vi "Multi RefTriggerScope with digital read long run.vi"() -> ()   [LabVIEW 2023]
uses:
  RefTriggerApplication/ApplicationCluster.ctl
  <instrlib>/niScope/Controls/niScope trigger source digital.ctl
  <instrlib>/niScope/Controls/niScope trigger slope.ctl
  <instrlib>/niDigital/niDigital.llb/niDigital Export Signal.ctl
  <instrlib>/niDigital/niDigital.llb/niDigital Trigger Digital Edge - Edge.ctl
  <instrlib>/niDigital/niDigital.llb/niDigital Trigger Terminals.ctl
  <instrlib>/niDCPower/nidcpower.llb/niDCPower Export Signal - Signal.ctl
  <instrlib>/niDCPower/nidcpower.llb/niDCPower Wait For Event - Event.ctl
  <instrlib>/niScope/Configure/Trigger/niScope Configure Trigger Digital.vi
  <instrlib>/niDigital/niDigital.llb/niDigital Disable Start Trigger.vi
  <instrlib>/niDigital/niDigital.llb/niDigital Write Source Waveform (Broadcast U32).vi
  <instrlib>/niDigital/niDigital.llb/niDigital Configure Digital Edge Start Trigger.vi
  <instrlib>/niScope/Acquire/Fetch/niScope Fetch.vi
  <vilib>/Utility/file.llb/Write Delimited Spreadsheet (DBL).vi
  <instrlib>/NIDigital Low-Level SPI/NIDigital Low-Level SPI.lvclass
  <instrlib>/niDigital/niDigital.llb/niDigital Burst Pattern (Pass Fail).vi
panel:
  in  "LoggingPath":path
  in  "Stop":bool
  out "SMU":dbl[](graph)
  in  "Trigger Through":enum16{"DigitalPattern", "SMU"}(ring)
  in  "Instrument Settings":enum32{"SMU", "Scope", "Digital Pattern"}(tab)
  in  "SMU name":refnum<k15>
  in  "Scope Name 2":refnum<k15>="Scope_5152_C02_S05" caption="Scope  Name(s)"
  in  "Scope Name":refnum<k15>="Scope_5152_C02_S05" caption="Scope  Name(s)"
  in  "Sample Rate":dbl=5000000.0 format="%#.2p"
  in  "Record Length":i32=10000 format="%.0p"
  in  "Reference Position":dbl=50.0 caption="Ref Position" format="%#.1f"
  in  "DigiPat name":refnum<k15>
  in  "pin list":string="SCLK_SPI, MOSI_SPI, MISO_SPI, CS_SPI"
  out "Scope":dbl[][](graph)
  out "Digital Data":u32[][](array[numeric]) format="%.0x"
  out "error out":errorcluster
  in  "error in":errorcluster
  # "SDA"
  # "Other pin"
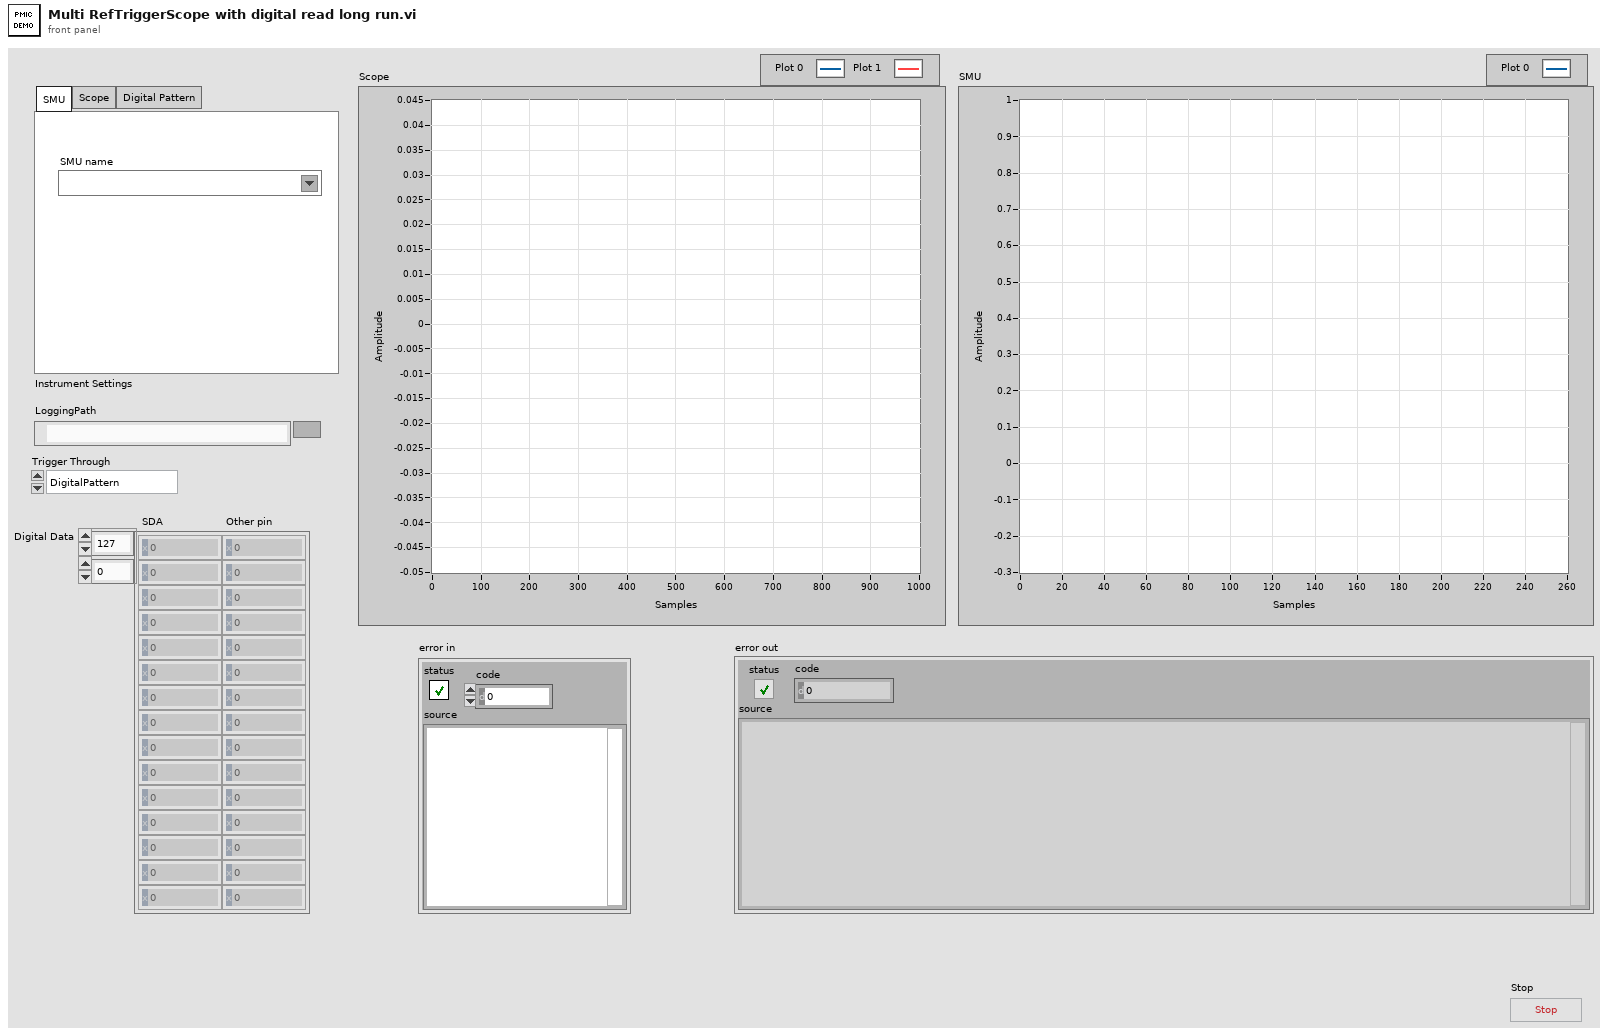
[diagram p1: front panel]
types:
  T1 = typedef "ApplicationCluster.ctl" = cluster{"Scope Name":refnum<k15>, "Scope channel name":string, "DigiPat name":refnum<k15>, "pin list":string, "DigitalWaveformName":string, "DigitalData":u32[][], "SMU name":refnum<k15>, "SMU Channel Name":string, "SMU Sequence Name":string, "Scope wfm":dbl[][], "SMU wfv":dbl[], "Record Length Scope":i32, "Scope Name 2":refnum<k15>, "Scope channel name 2":string}
  T2 = cluster{"Digital Data":u32[][], "SMU wfv":dbl[], "Scope wfm":dbl[][]}
  T3 = typedef "niScope trigger source digital.ctl" = string
  T4 = typedef "niDigital Trigger Terminals.ctl" = string
  T5 = typedef "niScope trigger slope.ctl" = i32
  T6 = typedef "niDigital Export Signal.ctl" = i32
  T7 = typedef "niDCPower Export Signal - Signal.ctl" = i32
  T8 = typedef "niDigital Trigger Digital Edge - Edge.ctl" = i32
  T9 = typedef "niDCPower Wait For Event - Event.ctl" = i32
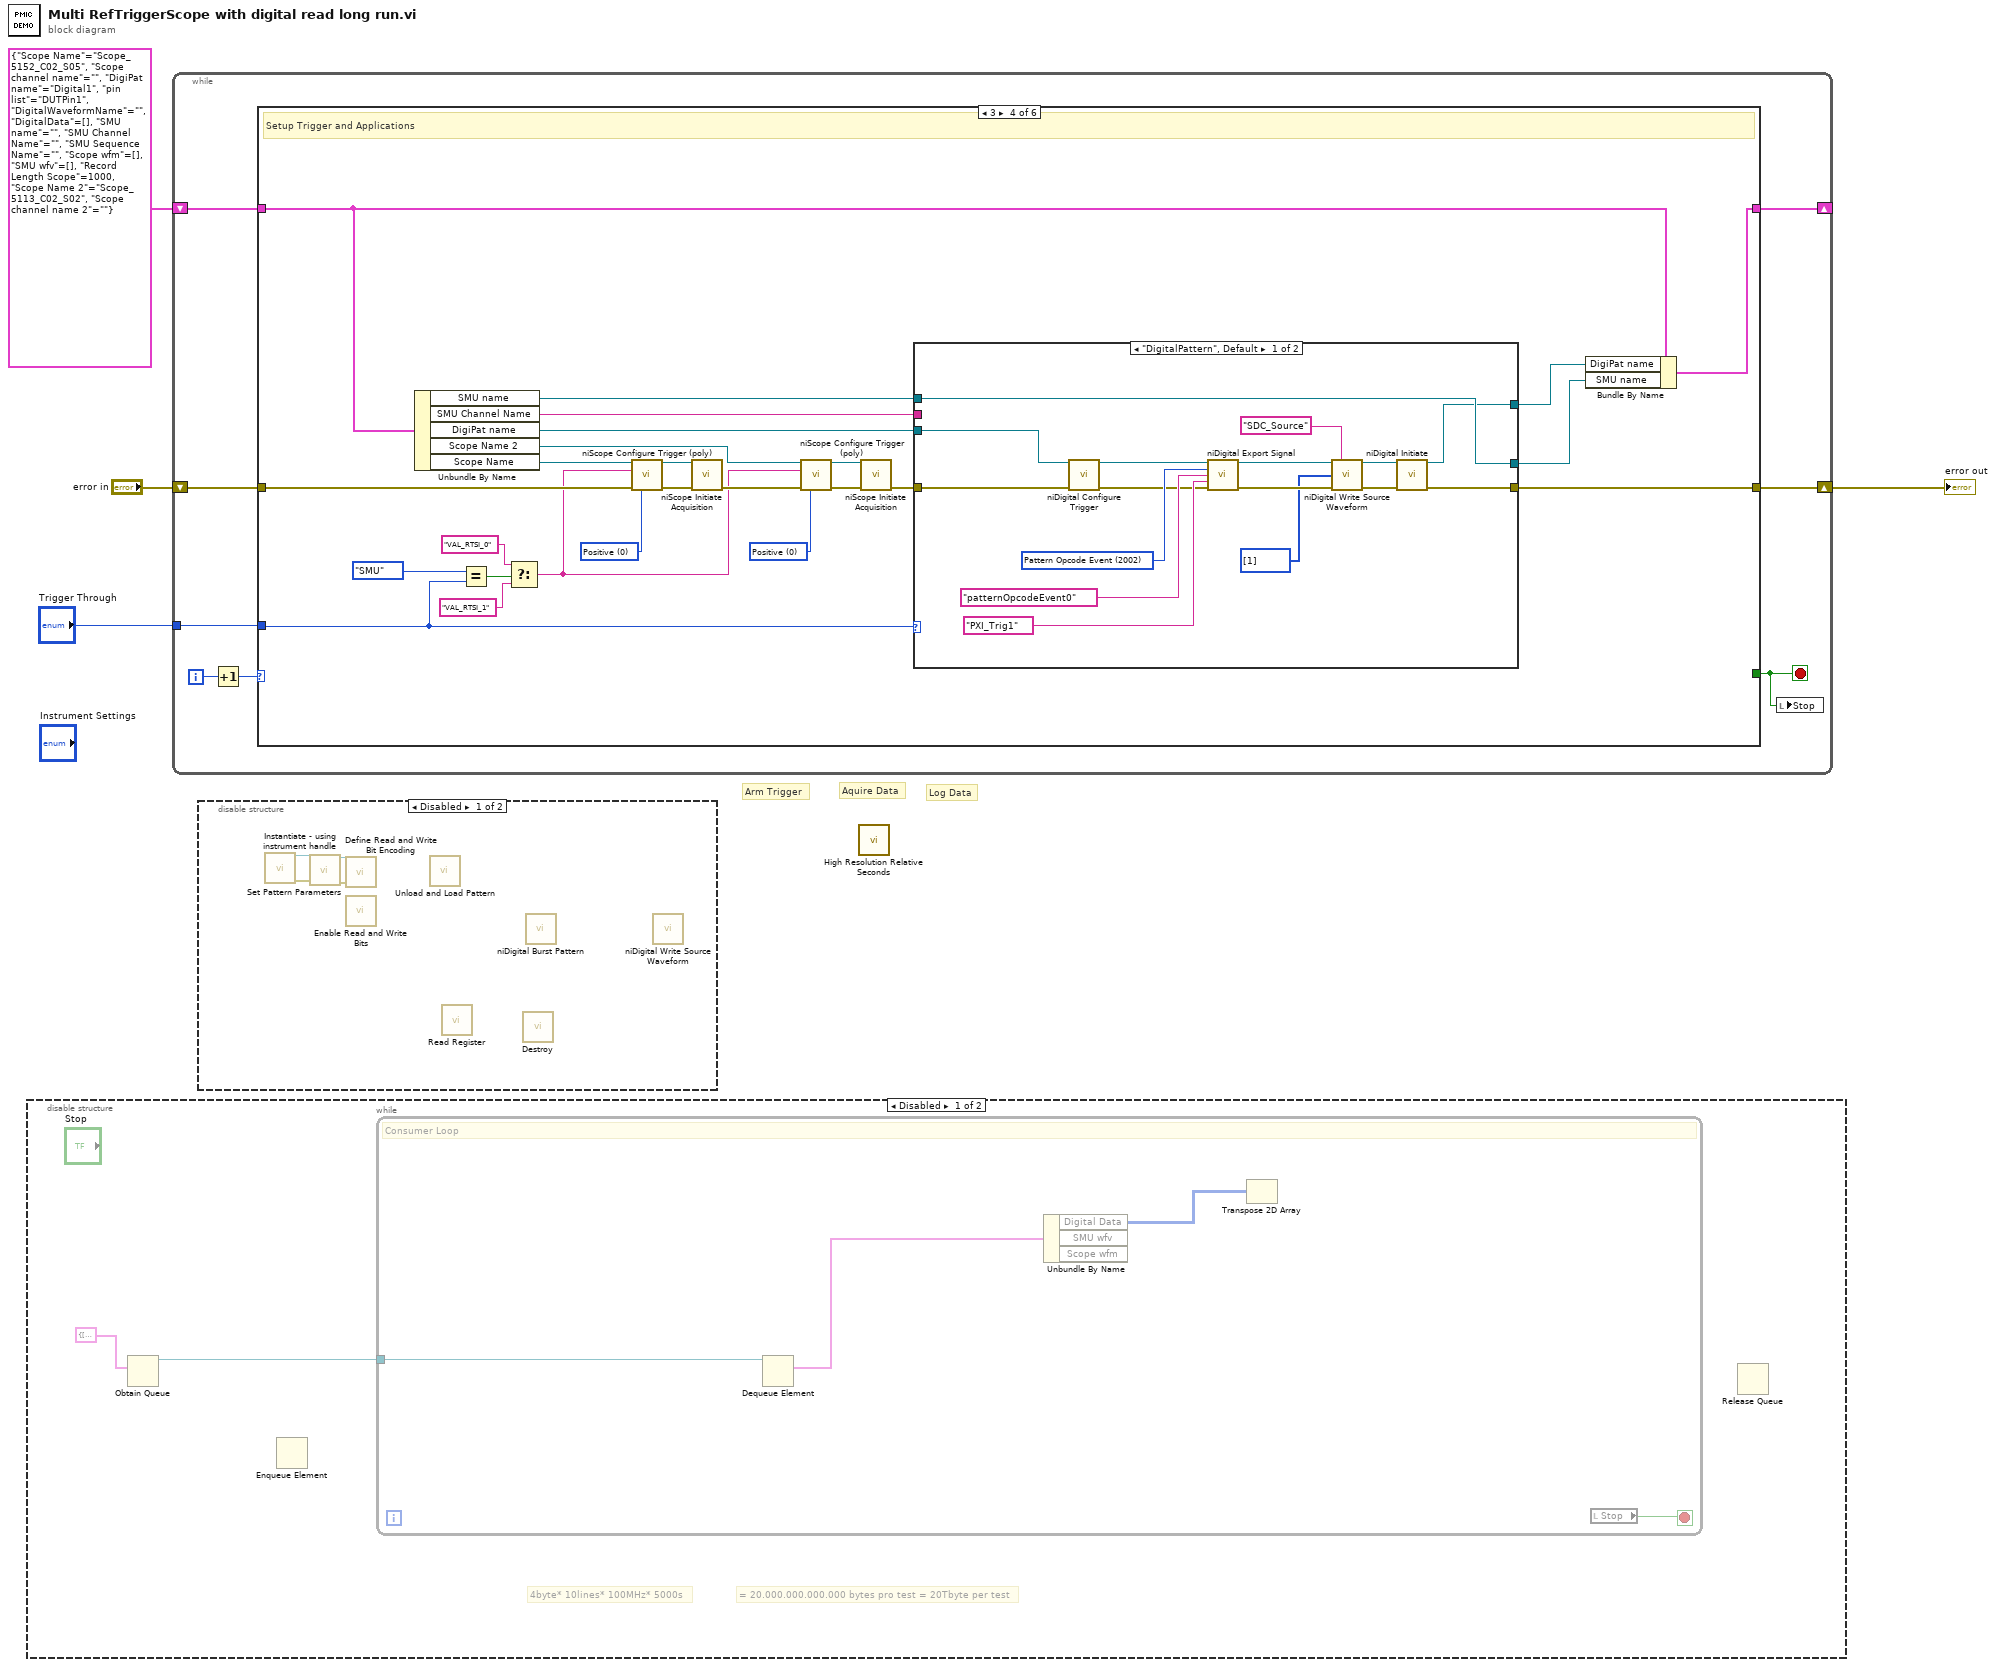
[diagram p0: block diagram]
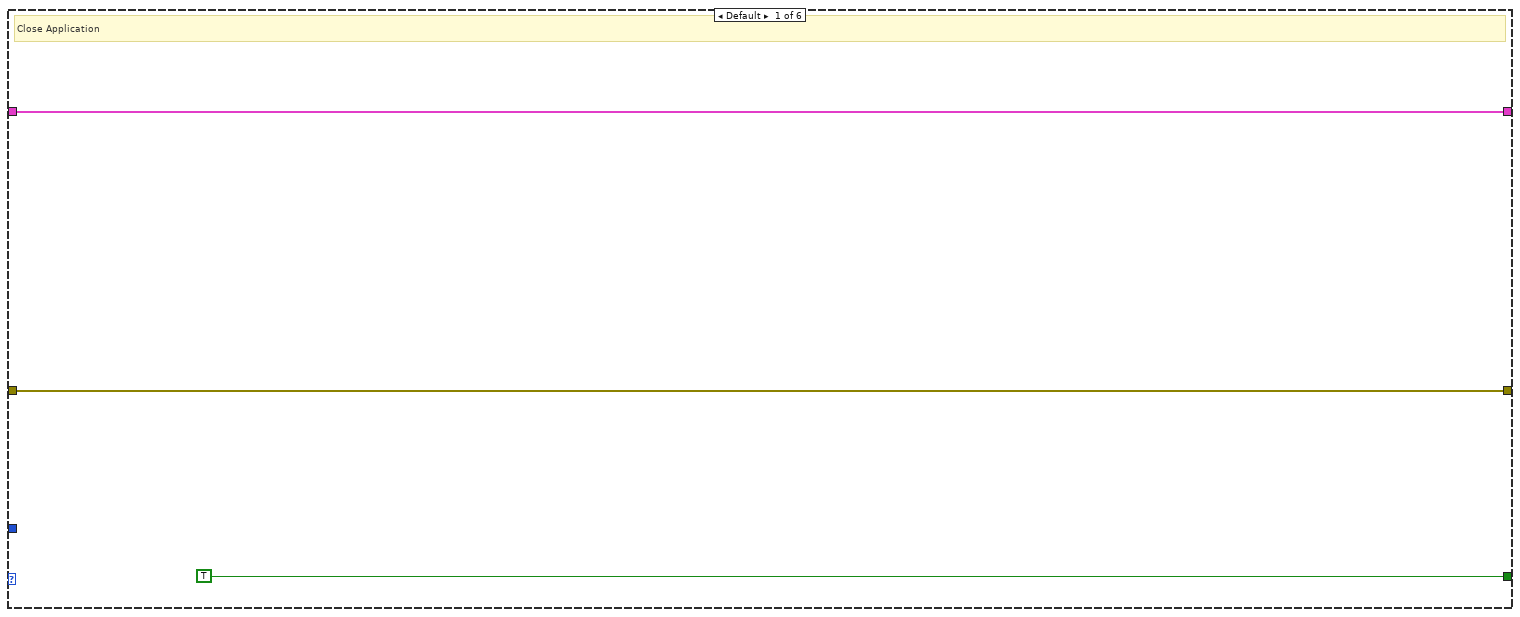
[diagram p4: hidden frame]
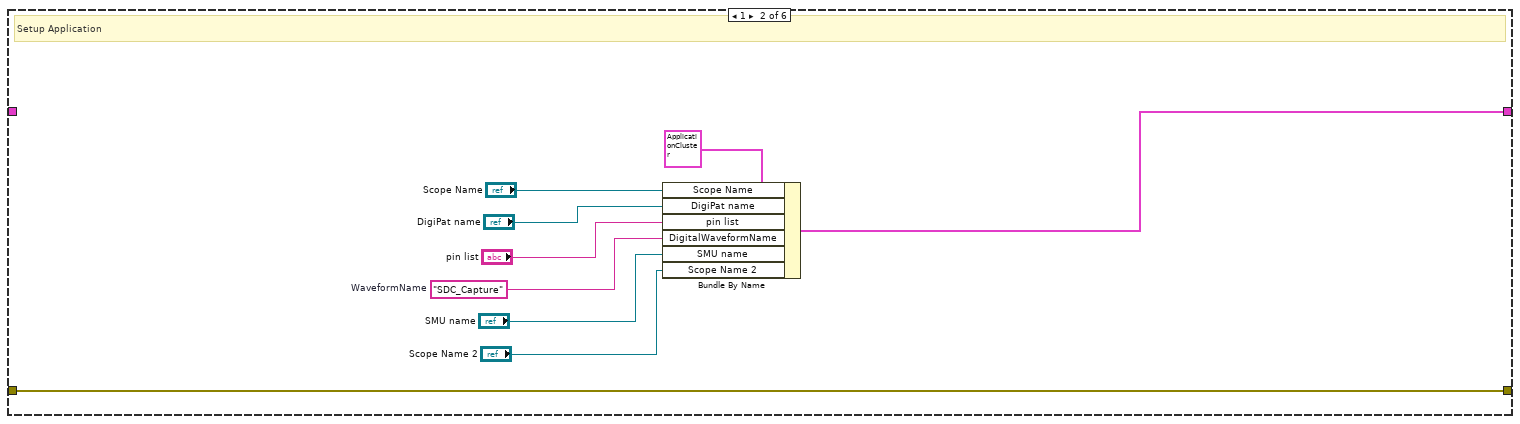
[diagram p5: hidden frame]
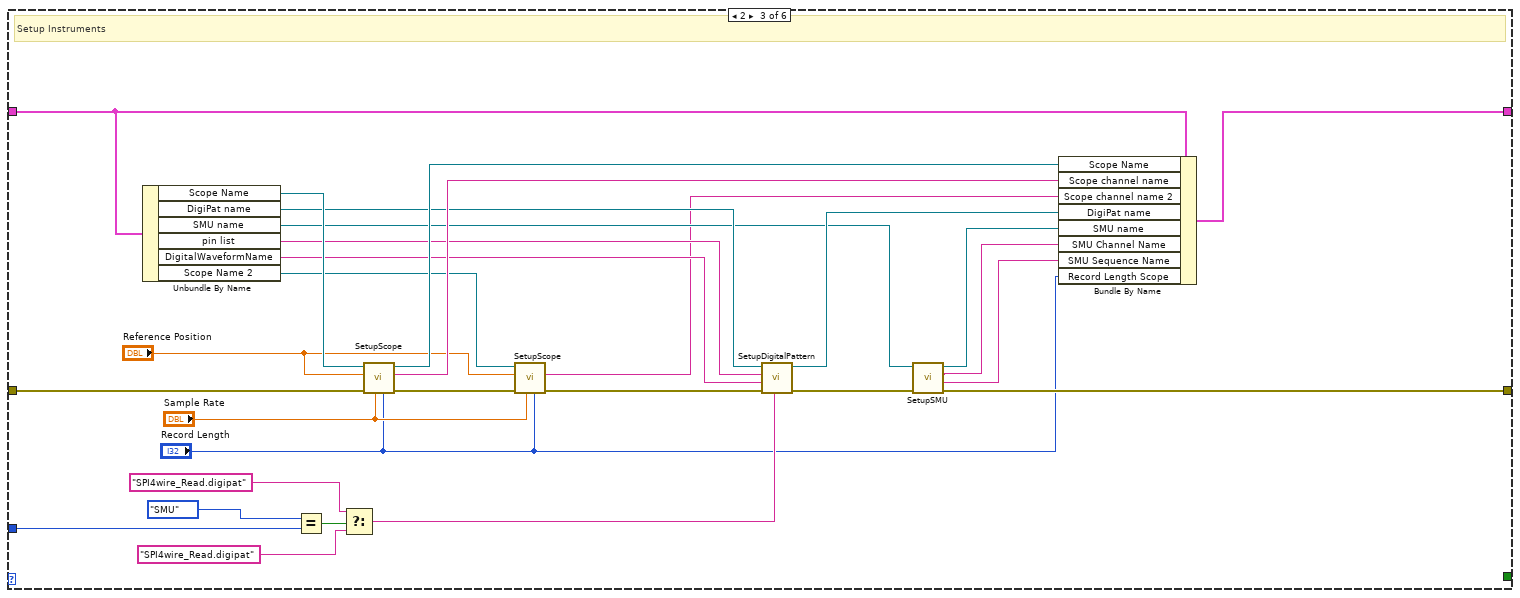
[diagram p6: hidden frame]
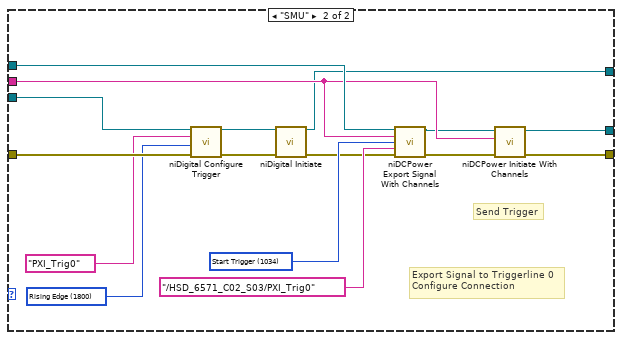
[diagram p7: hidden frame]
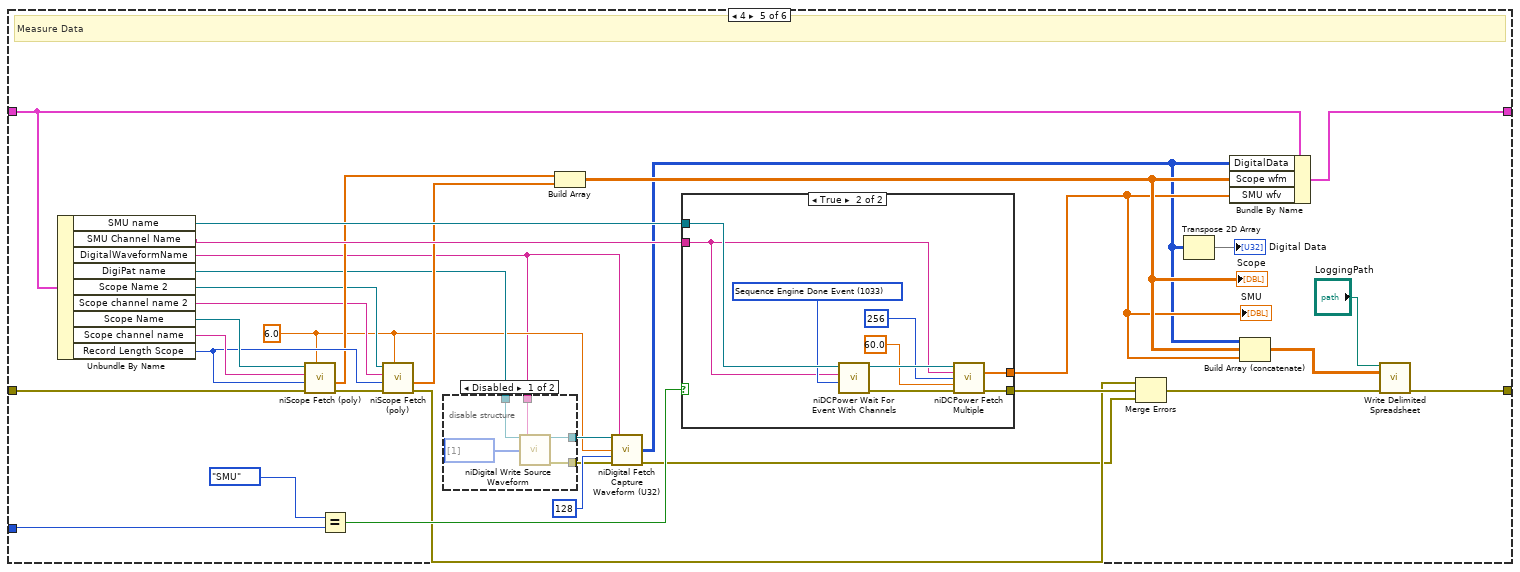
[diagram p8: hidden frame]
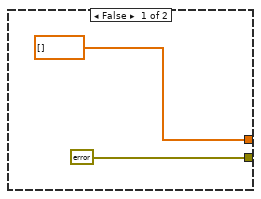
[diagram p10: hidden frame]
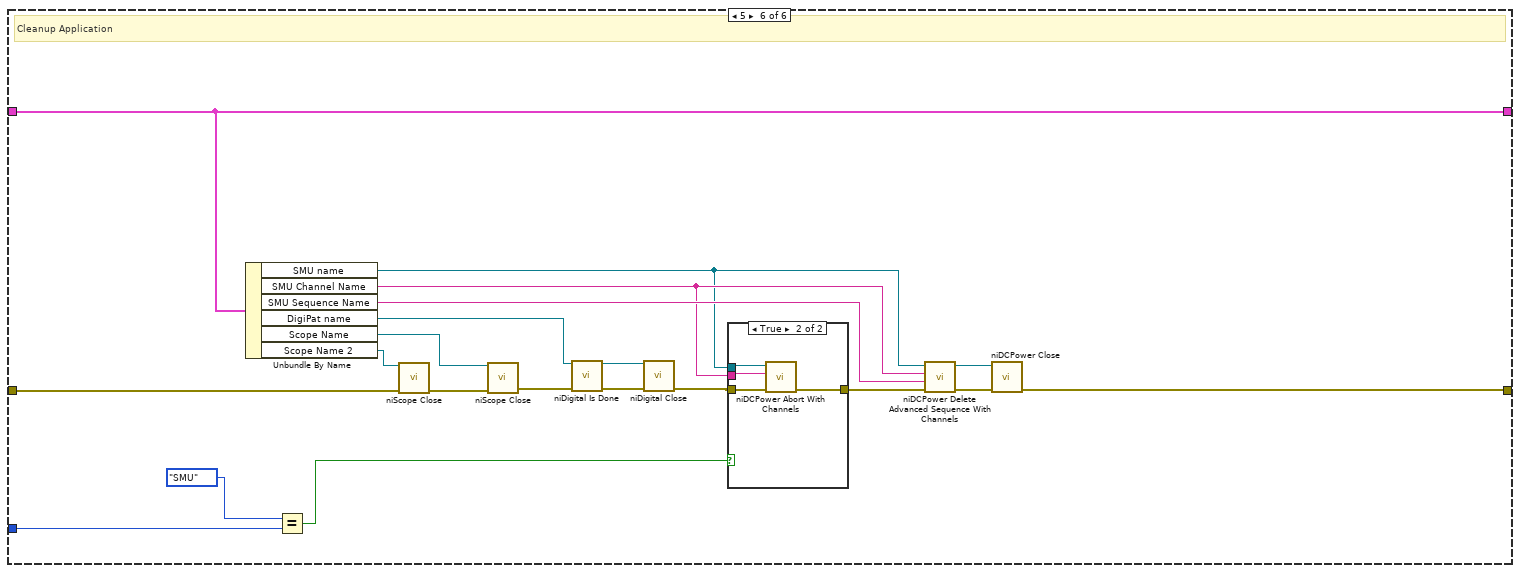
[diagram p11: hidden frame]
diagram:
  # "Log Data"
  # "Aquire Data"
  # "Arm Trigger"
  n1 = disable-structure shown="Disabled" {
    frame Disabled {
      # "= 20.000.000.000.000 bytes pro test = 20Tbyte per test"
      # "4byte* 10lines* 100MHz* 5000s"
      n2 = Obtain Queue(element data type=T2 {"Digital Data"=[], "SMU wfv"=[], "Scope wfm"=[]}) -> (queue out=w5:refnum<queue>)  [unwired: 4 in, 2 out]
      n3 = Enqueue Element() -> ()  [unwired: 4 in, 3 out]
      n4 = while {
        tunnel: w5 -> [w8]
        stop <- w10 stop-if-true
        # "Consumer Loop"
        n5 = Dequeue Element(queue=w8) -> (element=w7:T2)  [unwired: 2 in, 3 out]
        n6 = Unbundle By Name(w7) -> ("Digital Data"=w11:u32[][], "Scope wfm"=w9:dbl[][])  [unwired: 1 out]
        n7 = Transpose 2D Array(2D array=w11) -> ()  [unwired: 1 out]
        n8 = local read "Stop"() -> (w10:bool)
      }
      n9 = Release Queue() -> ()  [unwired: 3 in, 3 out]
    }
    frame Enabled {
    }
  }
  n10 = while {
    shift-right: [w19] -> w1
    shift-left: "error in" -> [w18]
    shift-right: [w17] -> _
    shift-left: T1 {"Scope Name"="Scope_5152_C02_S05", "Scope channel name"="", "DigiPat name"="Digital1", "pin list"="DUTPin1", "DigitalWaveformName"="", "DigitalData"=[], "SMU name"="", "SMU Channel Name"="", "SMU Sequence Name"="", "Scope wfm"=[], "SMU wfv"=[], "Record Length Scope"=1000, "Scope Name 2"="Scope_5113_C02_S02", "Scope channel name 2"=""} -> [w16]
    tunnel: "Trigger Through" -> [w13]
    i -> [w14]
    stop <- w12 stop-if-true
    n11 = Increment(x=w14) -> (x+1=w15:i32)
    n12 = case shown="3" w15 {
      tunnel: [w21 w28 w50 w80 w130 w185] -> w19
      tunnel: w18 -> [w21 w28 w60 w73 w150 w180]
      tunnel: [TRUE _ _ _ _ _] -> w12
      tunnel: [w20 w29 w56 w84 w148 w186] -> w17
      tunnel: w16 -> [w20 _ w58 w85 w149 w186]
      tunnel: w13 -> [_ _ w44 w70 w147 w169]
      frame Default {
        # "Close Application"
      }
      frame 1 {
        w25 = "SDC_Capture"  # WaveformName
        # "Setup Application"
        n13 = Bundle By Name(cluster=T1 {"Scope Name"="Scope_5152_C02_S05", "Scope channel name"="", "DigiPat name"="Digital1", "pin list"="DUTPin1", "DigitalWaveformName"="", "DigitalData"=[], "SMU name"="", "SMU Channel Name"="", "SMU Sequence Name"="", "Scope wfm"=[], "SMU wfv"=[], "Record Length Scope"=1000, "Scope Name 2"="Scope_5113_C02_S02", "Scope channel name 2"=""}, "Scope Name"="Scope Name", "DigiPat name"="DigiPat name", "pin list"="pin list", "DigitalWaveformName"=w25, "SMU name"="SMU name", "Scope Name 2"="Scope Name 2") -> (w29:T1)
      }
      frame 2 {
        # "Setup Instruments"
        n14 = Unbundle By Name(w58) -> ("Scope Name"=w59:refnum<k15>, "DigiPat name"=w54:refnum<k15>, "SMU name"=w51:refnum<k15>, "pin list"=w46:string, "DigitalWaveformName"=w45:string, "Scope Name 2"=w34:refnum<k15>)
        n15 = Equal?(x=enum16{"DigitalPattern", "SMU"}."SMU" ("Trigger Through"), y=w44) -> (x = y?=w43:bool)
        n16 = Select(t="SPI4wire_Read.digipat" ("PatternfileName"), s=w43, f="SPI4wire_Read.digipat") -> (s? t:f=w40:string)
        n17 = call "SetupScope.vi"("Record Length"="Record Length", "Sample Rate"="Sample Rate", "error in (no error)"=w60, "Reference Position"="Reference Position", "IVI Refnum in"=w59) -> ("error out"=w37:errorcluster, "channel name"=w55:string, "IVI Refnum out"=w57:refnum<k15>)  [unwired: 4 in]
        n18 = call "SetupScope.vi"("Record Length"="Record Length", "Sample Rate"="Sample Rate", "error in (no error)"=w37, "Reference Position"="Reference Position", "IVI Refnum in"=w34) -> ("error out"=w33:errorcluster, "channel name"=w32:string)  [unwired: 4 in, 1 out]
        n19 = call "SetupDigitalPattern.vi"("PatternfileName"=w40, "error in (no error)"=w33, "DigitalWaveformName"=w45, "pin list"=w46, "IVI Refnum in"=w54) -> ("error out"=w52:errorcluster, "IVI Refnum out"=w53:refnum<k15>)  [unwired: 5 in]
        n20 = call "SetupSMU.vi"("error in (no error)"=w52, "IVI Refnum in"=w51) -> ("error out"=w50:errorcluster, "SMU sequence name"=w47:string, "SMU Chanel Name"=w48:string, "instrument handle out"=w49:refnum<k15>)  [unwired: 6 in]
        n21 = Bundle By Name(cluster=w58, "Scope Name"=w57, "Scope channel name"=w55, "Scope channel name 2"=w32, "DigiPat name"=w53, "SMU name"=w49, "SMU Channel Name"=w48, "SMU Sequence Name"=w47, "Record Length Scope"="Record Length") -> (w56:T1)
      }
      frame 3 {
        w66 = T5 0 items=["Positive", "Negative"] ("trigger slope")
        w83 = T5 0 items=["Positive", "Negative"] ("trigger slope")
        # "Setup Trigger and Applications"
        n22 = Unbundle By Name(w85) -> ("SMU name"=w78:refnum<k15>, "SMU Channel Name"=w77:string, "DigiPat name"=w81:refnum<k15>, "Scope Name 2"=w61:refnum<k15>, "Scope Name"=w82:refnum<k15>)
        n23 = Equal?(x=enum16{"DigitalPattern", "SMU"}."SMU" ("Trigger Through"), y=w70) -> (x = y?=w72:bool)
        n24 = Select(t=T3 "VAL_RTSI_0" ("trigger source"), s=w72, f=T3 "VAL_RTSI_1" ("trigger source")) -> (s? t:f=w63:T3)
        n25 = call-poly <instrlib>:"niScope Configure Trigger (poly).vi"("instrument handle"=w82, "trigger slope"=w83, "trigger source"=w63, "error in"=w73) -> ("instrument handle out"=w74:refnum<k15>, "error out"=w75:errorcluster)  [unwired: 10 in]
        n26 = call <instrlib>:"niScope Initiate Acquisition.vi"("instrument handle"=w74, "error in"=w75) -> ("error out"=w65:errorcluster)  [unwired: 12 in, 1 out]
        n27 = call-poly <instrlib>:"niScope Configure Trigger (poly).vi"("instrument handle"=w61, "trigger slope"=w66, "trigger source"=w63, "error in"=w65) -> ("instrument handle out"=w62:refnum<k15>, "error out"=w67:errorcluster)  [unwired: 10 in]
        n28 = call <instrlib>:"niScope Initiate Acquisition.vi"("instrument handle"=w62, "error in"=w67) -> ("error out"=w64:errorcluster)  [unwired: 12 in, 1 out]
        n29 = case shown="\"DigitalPattern\", Default" w70 {
          tunnel: w64 -> [w92 w117]
          tunnel: w81 -> [w95 w116]
          tunnel: [w97 w111] -> w80
          tunnel: [w101 w110] -> w79
          tunnel: w78 -> [w101 w109]
          tunnel: w77 -> [_ w108]
          tunnel: [w96 w103] -> w76
          frame "DigitalPattern", Default {
            w100 = T6 2002 items=["Start Trigger"=2000, "Conditional Jump Trigger"=2001, "Pattern Opcode Event"=2002, "RIO Event"=2004] ("signal")
            n30 = call-poly <instrlib>:"niDigital Configure Trigger.vi"("instrument handle"=w95, "error in"=w92) -> ("instrument handle out"=w94:refnum<k15>, "error out"=w93:errorcluster)  [unwired: 12 in]
            n31 = call <instrlib>:"niDigital Export Signal.vi"("instrument handle"=w94, "signal"=w100, "signal ID"="patternOpcodeEvent0", "output terminal"="PXI_Trig1", "error in"=w93) -> ("instrument handle out"=w90:refnum<k15>, "error out"=w91:errorcluster)  [unwired: 9 in]
            n32 = call-poly <instrlib>:"niDigital Write Source Waveform.vi"("instrument handle"=w90, "waveform name"="SDC_Source", "waveform data"=u32[] [1], "error in"=w91) -> ("instrument handle out"=w89:refnum<k15>, "error out"=w88:errorcluster)  [unwired: 10 in]
            n33 = call <instrlib>:"niDigital Initiate.vi"("instrument handle"=w89, "error in"=w88) -> ("instrument handle out"=w96:refnum<k15>, "error out"=w97:errorcluster)  [unwired: 12 in]
          }
          frame "SMU" {
            w113 = T7 1034 items=["Source Complete Event"=1030, "Measure Complete Event"=1031, "Sequence Iteration Complete Event"=1032, "Sequence Engine Done Event"=1033, "Pulse Complete Event"=1051, "Ready For Pulse Trigger Event"=1052, "Start Trigger"=1034, "Source Trigger"=1035, "Measure Trigger"=1036, "Sequence Advance Trigger"=1037, "Pulse Trigger"=1053] ("signal")
            w115 = T8 1800 items=["Rising Edge"=1800, "Falling Edge"=1801] ("edge")
            # "Send Trigger"
            # "Export Signal to Triggerline 0\nConfigure Connection"
            n34 = call-poly <instrlib>:"niDigital Configure Trigger.vi"("instrument handle"=w116, "source"=T4 "PXI_Trig0", "edge"=w115, "error in"=w117) -> ("instrument handle out"=w106:refnum<k15>, "error out"=w107:errorcluster)  [unwired: 10 in]
            n35 = call <instrlib>:"niDigital Initiate.vi"("instrument handle"=w106, "error in"=w107) -> ("instrument handle out"=w103:refnum<k15>, "error out"=w105:errorcluster)  [unwired: 12 in]
            n36 = call <instrlib>:"niDCPower Export Signal With Channels.vi"("instrument handle"=w109, "channel name"=w108, "signal"=w113, "output terminal"=tag "/HSD_6571_C02_S03/PXI_Trig0", "error in (no error)"=w105) -> ("instrument handle out"=w102:refnum<k15>, "error out"=w104:errorcluster)  [unwired: 9 in]
            n37 = call <instrlib>:"niDCPower Initiate With Channels.vi"("error in (no error)"=w104, "channel name"=w108, "instrument handle"=w102) -> ("error out"=w111:errorcluster, "instrument handle out"=w110:refnum<k15>)  [unwired: 7 in]
          }
        }
        n38 = Bundle By Name(cluster=w85, "DigiPat name"=w76, "SMU name"=w79) -> (w84:T1)
      }
      frame 4 {
        w122 = 6.0 ("timeout")
        # "Measure Data"
        n39 = Unbundle By Name(w149) -> ("SMU name"=w144:refnum<k15>, "SMU Channel Name"=w143:string, "DigitalWaveformName"=w121:string, "DigiPat name"=w125:refnum<k15>, "Scope Name 2"=w134:refnum<k15>, "Scope channel name 2"=w133:string, "Scope Name"=w146:refnum<k15>, "Scope channel name"=w145:string, "Record Length Scope"=w137:i32)
        n40 = call-poly <instrlib>:"niScope Fetch (poly).vi"("timeout"=w122, "error in"=w150, "numSamples"=w137, "channels"=w145, "instrument handle"=w146) -> ("error out"=w138:errorcluster, "wfm"=w136:dbl[])  [unwired: 3 in, 2 out]
        n41 = Equal?(x=enum16{"DigitalPattern", "SMU"}."SMU" ("Trigger Through"), y=w147) -> (x = y?=w141:bool)
        n42 = call-poly <instrlib>:"niScope Fetch (poly).vi"("timeout"=w122, "error in"=w138, "numSamples"=w137, "channels"=w133, "instrument handle"=w134) -> ("error out"=w139:errorcluster, "wfm"=w135:dbl[])  [unwired: 3 in, 2 out]
        n43 = disable-structure shown="Disabled" {
          disable-tunnel: w125 -> [w155 w156]
          disable-tunnel: [w154 w156] -> w124
          disable-tunnel: w121 -> [w153 _]
          disable-tunnel: [w152 _] -> w120
          frame Disabled {
            n44 = call-poly <instrlib>:"niDigital Write Source Waveform.vi"("instrument handle"=w155, "waveform name"=w153, "waveform data"=u32[] [1]) -> ("instrument handle out"=w154:refnum<k15>, "error out"=w152:errorcluster)  [unwired: 11 in]
          }
          frame Enabled {
          }
        }
        n45 = Build Array(w136, w135) -> (w128:dbl[][])
        "Scope" <- w128
        n46 = call <instrlib>:"niDigital Fetch Capture Waveform (U32).vi"("instrument handle"=w124, "waveform name"=w121, "timeout (s)"=w122, "samples to read"=128, "error in"=w120) -> ("data"=w119:u32[][], "error out"=w118:errorcluster)  [unwired: 8 in, 1 out]
        n47 = case shown="True" w141 {
          tunnel: w144 -> [_ w165]
          tunnel: w143 -> [_ w163]
          tunnel: [errorcluster {"status"=FALSE, "code"=0, "source"=""} ("error out") w162] -> w142
          tunnel: [dbl[] [] ("voltage measurements") w161] -> w127
          frame False {
          }
          frame True {
            w164 = T9 1033 items=["Source Complete Event"=1030, "Measure Complete Event"=1031, "Sequence Iteration Complete Event"=1032, "Sequence Engine Done Event"=1033, "Pulse Complete Event"=1051, "Ready For Pulse Trigger Event"=1052] ("event")
            n48 = call <instrlib>:"niDCPower Wait For Event With Channels.vi"("event"=w164, "channel name"=w163, "instrument handle"=w165) -> ("error out"=w166:errorcluster, "instrument handle out"=w167:refnum<k15>)  [unwired: 7 in]
            n49 = call <instrlib>:"niDCPower Fetch Multiple.vi"("instrument handle"=w167, "channel name"=w163, "count (1)"=256 ("numSamples"), "timeout (1.0)"=60.0, "error in (no error)"=w166) -> ("voltage measurements"=w161:dbl[], "error out"=w162:errorcluster)  [unwired: 5 in, 4 out]
          }
        }
        "SMU" <- w127
        n50 = Merge Errors(w139, w142, w118) -> (w131:errorcluster)
        n51 = Transpose 2D Array(2D array=w119) -> (transposed array=→"Digital Data":u32[][])
        n52 = Bundle By Name(cluster=w149, "DigitalData"=w119, "Scope wfm"=w128, "SMU wfv"=w127) -> (w148:T1)
        n53 = Build Array (concatenate)(w119, w128, w127) -> (w126:dbl[][])
        n54 = call-poly <vilib>:"Write Delimited Spreadsheet.vi"("file path (dialog if empty)"="LoggingPath", "2D data"=w126, "error in (no error)"=w131) -> ("error out"=w130:errorcluster)  [unwired: 11 in, 1 out]
      }
      frame 5 {
        # "Cleanup Application"
        n55 = Unbundle By Name(w186) -> ("SMU name"=w175:refnum<k15>, "SMU Channel Name"=w176:string, "SMU Sequence Name"=w182:string, "DigiPat name"=w172:refnum<k15>, "Scope Name"=w187:refnum<k15>, "Scope Name 2"=w181:refnum<k15>)
        n56 = Equal?(x=enum16{"DigitalPattern", "SMU"}."SMU" ("Trigger Through"), y=w169) -> (x = y?=w168:bool)
        n57 = call <instrlib>:"niScope Close.vi"("instrument handle"=w181, "error in"=w180) -> ("error out"=w179:errorcluster)  [unwired: 13 in]
        n58 = call <instrlib>:"niScope Close.vi"("instrument handle"=w187, "error in"=w179) -> ("error out"=w173:errorcluster)  [unwired: 13 in]
        n59 = call <instrlib>:"niDigital Is Done.vi"("instrument handle"=w172, "error in"=w173) -> ("instrument handle out"=w171:refnum<k15>, "error out"=w178:errorcluster)  [unwired: 11 in, 1 out]
        n60 = call <instrlib>:"niDigital Close.vi"("instrument handle"=w171, "error in"=w178) -> ("error out"=w177:errorcluster)  [unwired: 13 in]
        n61 = case shown="True" w168 {
          tunnel: w177 -> [w188 w192]
          tunnel: w176 -> [_ w191]
          tunnel: w175 -> [_ w190]
          tunnel: [w188 w189] -> w174
          frame False {
          }
          frame True {
            n62 = call <instrlib>:"niDCPower Abort With Channels.vi"("error in (no error)"=w192, "channel name"=w191, "instrument handle"=w190) -> ("error out"=w189:errorcluster)  [unwired: 7 in, 1 out]
          }
        }
        n63 = call <instrlib>:"niDCPower Delete Advanced Sequence With Channels.vi"("error in (no error)"=w174, "sequence name"=w182, "channel name"=w176, "instrument handle"=w175) -> ("error out"=w184:errorcluster, "instrument handle out"=w183:refnum<k15>)  [unwired: 6 in]
        n64 = call <instrlib>:"niDCPower Close.vi"("error in (no error)"=w184, "instrument handle"=w183) -> ("error out"=w185:errorcluster)  [unwired: 9 in]
      }
    }
    n65 = local write "Stop"(w12) -> ()
  }
  "error out" <- w1
  n66 = disable-structure shown="Disabled" {
    frame Disabled {
      n67 = call <instrlib>:"Instantiate - using instrument handle.vi"() -> ("NIDigital Low Level SPI out"=w196:refnum<class "NIDigital Low-Level SPI.lvclass">, "error out"=w195:errorcluster)  [unwired: 14 in]
      n68 = call <instrlib>:"Set Pattern Parameters.vi"("NIDigital Low Level SPI in"=w196, "error in (no error)"=w195) -> ("NIDigital Low Level SPI out"=w194:refnum<class "NIDigital Low-Level SPI.lvclass">, "error out"=w193:errorcluster)  [unwired: 12 in]
      n69 = call <instrlib>:"Define Read and Write Bit Encoding.vi"("NIDigital Low Level SPI in"=w194, "error in (no error)"=w193) -> ()  [unwired: 12 in, 2 out]
      n70 = call <instrlib>:"Enable Read and Write Bits.vi"() -> ()  [unwired: 14 in, 2 out]
      n71 = call <instrlib>:"Unload and Load Pattern.vi"() -> ()  [unwired: 14 in, 2 out]
      n72 = call <instrlib>:"Read Register.vi"() -> ()  [unwired: 13 in, 3 out]
      n73 = call <instrlib>:"Destroy.vi"() -> ()  [unwired: 14 in, 2 out]
      n74 = call-poly <instrlib>:"niDigital Burst Pattern.vi"() -> ()  [unwired: 13 in, 3 out]
      n75 = call-poly <instrlib>:"niDigital Write Source Waveform.vi"() -> ()  [unwired: 14 in, 2 out]
    }
    frame Enabled {
    }
  }
  n76 = call <vilib>:"High Resolution Relative Seconds.vi"() -> ()  [unwired: 1 out]
